vi "solar_excel Worksheet Close.vi"(8 "error in (no error)":errorcluster, 11 "Excel Worksheet":T2) -> (0 "error out":errorcluster, 3 "Excel Workbook":T1)   [LabVIEW 2018]
doc: "This closes a Worksheet reference and returns the Workbook reference."
uses:
  solar_excel_ctl Workbook.ctl
  solar_excel_ctl TSV.ctl
  solar_excel_ctl Worksheet.ctl
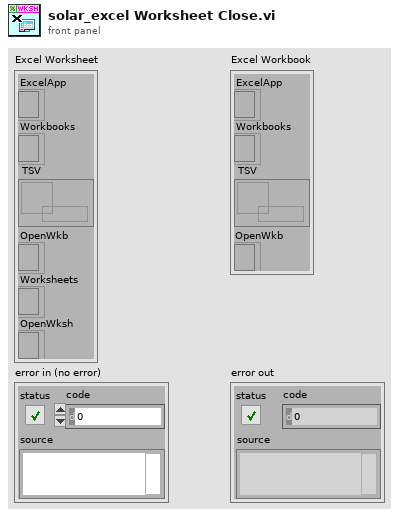
[diagram p1: front panel]
types:
  T1 = typedef "solar_excel_ctl Workbook.ctl" = cluster{"ExcelApp":refnum<k7>, "Workbooks":refnum<k7>, "TSV":refnum<queue>, "OpenWkb":refnum<k7>}
  T2 = typedef "solar_excel_ctl Worksheet.ctl" = cluster{"ExcelApp":refnum<k7>, "Workbooks":refnum<k7>, "TSV":refnum<queue>, "OpenWkb":refnum<k7>, "Worksheets":refnum<k7>, "OpenWksh":refnum<k7>}
  T3 = typedef "solar_excel_ctl TSV.ctl" = cluster{"Path":path, "Dirty":bool, "ActiveSheet":u8, "Worksheets":string[], "Worksheet Cells":cluster{"Cells":string[][]}[]}
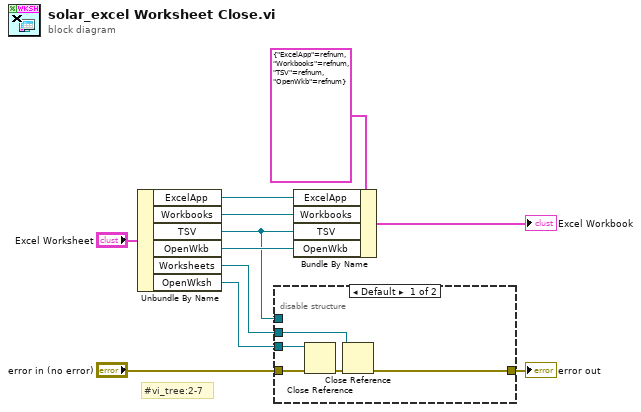
[diagram p0: block diagram]
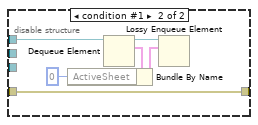
[diagram p2: hidden frame]
diagram:
  # "#vi_tree:2-7"
  n1 = Unbundle By Name("Excel Worksheet") -> ("ExcelApp"=w11:refnum<k7>, "Workbooks"=w10:refnum<k7>, "TSV"=w1:refnum<queue>, "OpenWkb"=w9:refnum<k7>, "Worksheets"=w2:refnum<k7>, "OpenWksh"=w6:refnum<k7>)
  n2 = disable-structure shown="Default" {
    disable-tunnel: "error in (no error)" -> [w16 w17]
    disable-tunnel: w6 -> [w15 _]
    disable-tunnel: [w13 w17] -> w3
    disable-tunnel: w2 -> [w12 _]
    disable-tunnel: w1 -> [_ w22]
    frame condition #0 (active) {
      n3 = Close Reference(reference=w15, error in (no error)=w16) -> (error out=w14:errorcluster)
      n4 = Close Reference(reference=w12, error in (no error)=w14) -> (error out=w13:errorcluster)
    }
    frame condition #1 {
      n5 = Dequeue Element(queue=w22) -> (queue out=w21:refnum<queue>, element=w20:T3)  [unwired: 2 in, 2 out]
      n6 = Bundle By Name(cluster=w20, "ActiveSheet"=u8 0) -> (w19:T3)
      n7 = Lossy Enqueue Element(queue=w21, element=w19) -> ()  [unwired: 1 in, 4 out]
    }
  }
  "error out" <- w3
  n8 = Bundle By Name(cluster=T1 {"ExcelApp"=refnum, "Workbooks"=refnum, "TSV"=refnum, "OpenWkb"=refnum} ("Excel Workbook"), "ExcelApp"=w11, "Workbooks"=w10, "TSV"=w1, "OpenWkb"=w9) -> (→"Excel Workbook":T1)
